vi "_PC_Daemon_Pref init_ion_sources_interface.vi"(7 "eng_mode_str":refnum<vi>, 8 "error in (no error)":errorcluster, 9 "DI Array":refnum<vi>[](array[refnum]), 10 "DO Array":refnum<vi>[](array[refnum]), 11 "AO Array":refnum<vi>[](array[refnum])) -> (0 "error out":errorcluster, 1 "DI Array out":refnum<vi>[](array[refnum]), 2 "DO Array out":refnum<vi>[](array[refnum]), 3 "AO Array out":refnum<vi>[](array[refnum]))   [LabVIEW 2018]
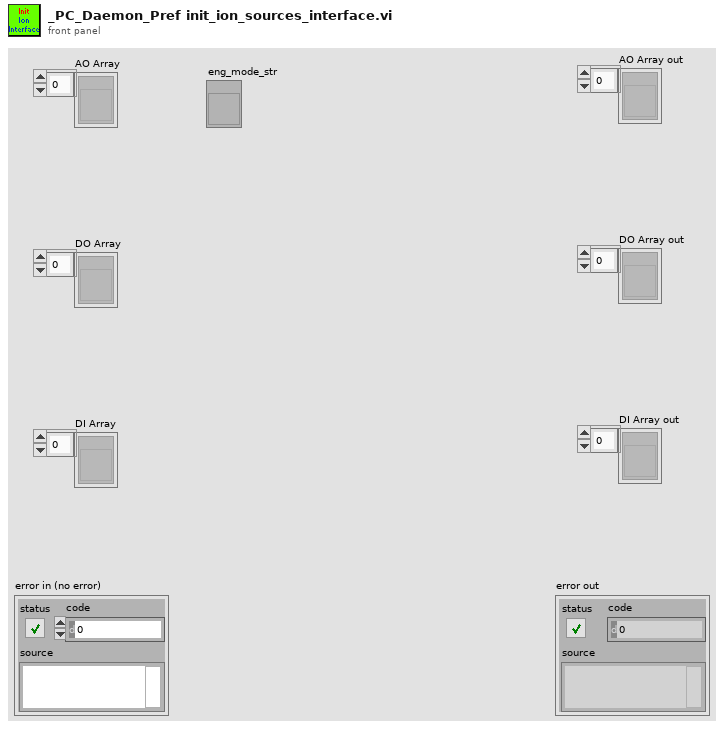
[diagram p1: front panel]
types:
  T1 = enum8{"Enabled", "Disabled", "Disabled and Grayed Out"}
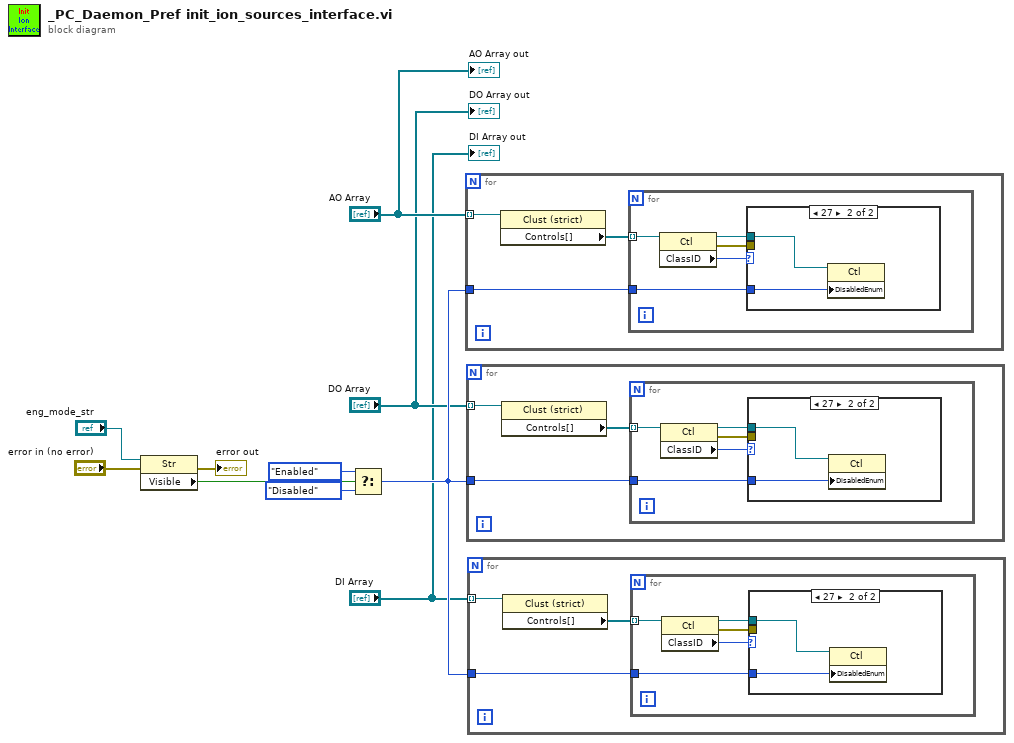
[diagram p0: block diagram]
diagram:
  n1 = property class="Str"(reference="eng_mode_str", error in="error in (no error)") -> (error out=→"error out":errorcluster, "Visible"=w9:bool)  [unwired: 1 out]
  n2 = Select(t=T1."Enabled" ("Disabled"), s=w9, f=T1."Disabled" ("Disabled")) -> (s? t:f=w6:T1)
  n3 = for {
    tunnel: "AO Array" -> [w13] mode=indexing
    tunnel: w6 -> [w11]
    n4 = property class="Clust (strict)"(reference=w13) -> ("Controls[]"=w12:refnum<vi>[])  [unwired: 1 in, 2 out]
    n5 = for {
      tunnel: w12 -> [w18] mode=indexing
      tunnel: w11 -> [w14]
      n6 = property class="Ctl"(reference=w18) -> (reference out=w16:refnum<vi>, error out=w15:errorcluster, "ClassID"=w17:u32)  [unwired: 1 in]
      n7 = case shown="27" w17 {
        tunnel: w16 -> [_ w20]
        tunnel: w15 -> [_ _]
        tunnel: w14 -> [_ w19]
        frame 0, Default {
        }
        frame 27 {
          n8 = property class="Ctl"(reference=w20, "DisabledEnum"=w19) -> ()  [unwired: 1 in, 2 out]
        }
      }
    }
  }
  n9 = for {
    tunnel: "DO Array" -> [w23] mode=indexing
    tunnel: w6 -> [w21]
    n10 = property class="Clust (strict)"(reference=w23) -> ("Controls[]"=w22:refnum<vi>[])  [unwired: 1 in, 2 out]
    n11 = for {
      tunnel: w22 -> [w28] mode=indexing
      tunnel: w21 -> [w24]
      n12 = property class="Ctl"(reference=w28) -> (reference out=w26:refnum<vi>, error out=w25:errorcluster, "ClassID"=w27:u32)  [unwired: 1 in]
      n13 = case shown="27" w27 {
        tunnel: w26 -> [_ w30]
        tunnel: w25 -> [_ _]
        tunnel: w24 -> [_ w29]
        frame 0, Default {
        }
        frame 27 {
          n14 = property class="Ctl"(reference=w30, "DisabledEnum"=w29) -> ()  [unwired: 1 in, 2 out]
        }
      }
    }
  }
  n15 = for {
    tunnel: "DI Array" -> [w33] mode=indexing
    tunnel: w6 -> [w31]
    n16 = property class="Clust (strict)"(reference=w33) -> ("Controls[]"=w32:refnum<vi>[])  [unwired: 1 in, 2 out]
    n17 = for {
      tunnel: w32 -> [w38] mode=indexing
      tunnel: w31 -> [w34]
      n18 = property class="Ctl"(reference=w38) -> (reference out=w36:refnum<vi>, error out=w35:errorcluster, "ClassID"=w37:u32)  [unwired: 1 in]
      n19 = case shown="27" w37 {
        tunnel: w36 -> [_ w40]
        tunnel: w35 -> [_ _]
        tunnel: w34 -> [_ w39]
        frame 0, Default {
        }
        frame 27 {
          n20 = property class="Ctl"(reference=w40, "DisabledEnum"=w39) -> ()  [unwired: 1 in, 2 out]
        }
      }
    }
  }
  "AO Array out" <- "AO Array"
  "DO Array out" <- "DO Array"
  "DI Array out" <- "DI Array"
